vi "TangentLineAngle.vi"(1 "Radius":dbl, 2 "DestPoint":T1) -> (0 "Tangent Angle Offset (rad)":dbl)   [LabVIEW 2017]
uses:
  PathPlanning/TypeDefs/Point2D.ctl
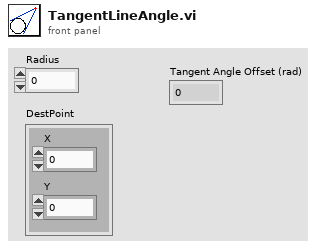
[diagram p1: front panel]
types:
  T1 = typedef "Point2D.ctl" = cluster{"X":dbl, "Y":dbl}
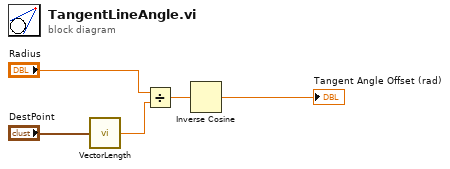
[diagram p0: block diagram]
diagram:
  n1 = call "VectorLength.vi"("VectorIn"="DestPoint") -> ("VectorLength"=w1:dbl)
  n2 = Divide(x="Radius", y=w1) -> (x/y=w4:dbl)
  n3 = Inverse Cosine(1:w4) -> (0:→"Tangent Angle Offset (rad)":dbl)
